vi "main(Test DQMH modules).vi"() -> ()   [LabVIEW 2018, in "Application.lvlib"] (continued)
        n3743 = Flush Queue(queue=w8192) -> (queue out=w8184:refnum<queue>)  [unwired: 1 in, 2 out]
        n3744 = Decrement(x=w8179) -> (x-1=w8183:i32)
        n3745 = Index Array(array=w8180, index=w8183) -> (element=w8181:refnum<vi>)
        n3746 = property class="ColBox"(reference=w8181, "Value"=u32 10000536 ("DRV 1")) -> ()  [unwired: 1 in, 2 out]
        n3747 = To Variant(anything=bool[] [FALSE, TRUE, FALSE, FALSE, FALSE, FALSE]) -> (Variant=w8209:variant)
        n3748 = To Variant(anything=T6."demux1_10_channel7" ("demux1_10(x6)_encode")) -> (Variant=w8213:variant)
        n3749 = To Variant(anything=T4."mux6_1_channel2_3" ("mux6_1(3wires)_encode")) -> (Variant=w8216:variant)
        n3750 = To Variant(anything=T5."mux10_1_channel7" ("mux10_1(x6)_encode")) -> (Variant=w8218:variant)
        n3751 = Bundle By Name(cluster=w8212, "command"="MEAS.mux10-1", "command data"=w8218) -> (w8207:T11)
        n3752 = Bundle By Name(cluster=w8212, "command"="MEAS.mux6_1", "command data"=w8216) -> (w8206:T11)
        n3753 = Bundle By Name(cluster=w8212, "command"="MEAS.demux1-10", "command data"=w8213) -> (w8205:T11)
        n3754 = Bundle By Name(cluster=w8212, "command"="MEAS.eMIC", "command data"=w8209) -> (w8204:T11)
        n3755 = Bundle By Name(cluster=w8212, "command"="MEAS.AllRelaysOFF") -> (w8208:T11)
        n3756 = Build Array(w8208, w8207, w8206, w8205, w8204) -> (w8199:T11[])
        n3757 = Bundle By Name(cluster=w8187, "command"="MEAS.requestAC", "command data"=w8179) -> (w8200:T11)
        n3758 = Bundle By Name(cluster=w8187, "command"="Apps.WaitForEvent", "command data"=w8179) -> (w8186:T11)
        n3759 = Bundle By Name(cluster=w8187, "command"="MEAS.DMM dual read") -> (w8201:T11)
        n3760 = Bundle By Name(cluster=w8187, "command"="Apps.UI Update 1") -> (w8188:T11)
        n3761 = Build Array(w8201, w8200, w8186, w8188) -> (w8198:T11[])
        n3762 = Build Array (concatenate)(w8199, w8198) -> (w8197:T11[])
        n3763 = for {
          tunnel: w8197 -> [w8234] mode=indexing
          tunnel: w8184 -> [w8235]
          tunnel: [w8231] -> w8195 mode=indexing
          n3764 = Unbundle By Name(w8234) -> ("command"=w8233:string, "command data"=w8232:variant)
          n3765 = call "App enquece.vi"("command data"=w8232, "command"=w8233, "queue in"=w8235) -> ("error out"=w8231:errorcluster)  [unwired: 7 in, 1 out]
        }
        n3766 = Merge Errors(w8196, w8195) -> (w8194:errorcluster)
      }
      frame "Test DRV 39A" {
        w8243 = T11 {"command"="", "command data"=variant} ("element")
        w8236 = 39 ("DUT index(0-59)")
        w8269 = T11 {"command"="", "command data"=variant} ("element")
        n3767 = disable-structure shown="LOGGING==TRUE" {
          disable-tunnel: w8247 -> [w8284 _]
          frame condition #0 (active) {
            n3768 = Empty String/Path?(string/path=w8284) -> (empty?=w8287:bool)
            n3769 = Select(t="Quece timeout", s=w8287, f=w8284) -> (s? t:f=w8283:string)
            n3770 = call "string log (SubVI).vi"("Enum"=enum16{"Init", "Log", "Read"}."Log", "state Name"=w8283) -> ()  [unwired: 8 in, 2 out]
          }
          frame condition #1 {
          }
        }
        n3771 = Flush Queue(queue=w8248) -> (queue out=w8249:refnum<queue>)  [unwired: 1 in, 2 out]
        n3772 = Decrement(x=w8236) -> (x-1=w8240:i32)
        n3773 = Index Array(array=w8237, index=w8240) -> (element=w8238:refnum<vi>)
        n3774 = property class="ColBox"(reference=w8238, "Value"=u32 10000536 ("DRV 1")) -> ()  [unwired: 1 in, 2 out]
        n3775 = To Variant(anything=bool[] [FALSE, FALSE, TRUE, FALSE, FALSE, FALSE]) -> (Variant=w8266:variant)
        n3776 = To Variant(anything=T6."demux1_10_channel7" ("demux1_10(x6)_encode")) -> (Variant=w8270:variant)
        n3777 = To Variant(anything=T4."mux6_1_channel3_3" ("mux6_1(3wires)_encode")) -> (Variant=w8273:variant)
        n3778 = To Variant(anything=T5."mux10_1_channel7" ("mux10_1(x6)_encode")) -> (Variant=w8275:variant)
        n3779 = Bundle By Name(cluster=w8269, "command"="MEAS.mux10-1", "command data"=w8275) -> (w8264:T11)
        n3780 = Bundle By Name(cluster=w8269, "command"="MEAS.mux6_1", "command data"=w8273) -> (w8263:T11)
        n3781 = Bundle By Name(cluster=w8269, "command"="MEAS.demux1-10", "command data"=w8270) -> (w8262:T11)
        n3782 = Bundle By Name(cluster=w8269, "command"="MEAS.eMIC", "command data"=w8266) -> (w8261:T11)
        n3783 = Bundle By Name(cluster=w8269, "command"="MEAS.AllRelaysOFF") -> (w8265:T11)
        n3784 = Build Array(w8265, w8264, w8263, w8262, w8261) -> (w8256:T11[])
        n3785 = Bundle By Name(cluster=w8243, "command"="MEAS.requestAC", "command data"=w8236) -> (w8257:T11)
        n3786 = Bundle By Name(cluster=w8243, "command"="Apps.WaitForEvent", "command data"=w8236) -> (w8242:T11)
        n3787 = Bundle By Name(cluster=w8243, "command"="MEAS.DMM dual read") -> (w8258:T11)
        n3788 = Bundle By Name(cluster=w8243, "command"="Apps.UI Update 1") -> (w8244:T11)
        n3789 = Build Array(w8258, w8257, w8242, w8244) -> (w8255:T11[])
        n3790 = Build Array (concatenate)(w8256, w8255) -> (w8254:T11[])
        n3791 = for {
          tunnel: w8254 -> [w8291] mode=indexing
          tunnel: w8249 -> [w8292]
          tunnel: [w8288] -> w8252 mode=indexing
          n3792 = Unbundle By Name(w8291) -> ("command"=w8290:string, "command data"=w8289:variant)
          n3793 = call "App enquece.vi"("command data"=w8289, "command"=w8290, "queue in"=w8292) -> ("error out"=w8288:errorcluster)  [unwired: 7 in, 1 out]
        }
        n3794 = Merge Errors(w8253, w8252) -> (w8251:errorcluster)
      }
      frame "Test DRV 40A" {
        w8300 = T11 {"command"="", "command data"=variant} ("element")
        w8293 = 40 ("DUT index(0-59)")
        w8326 = T11 {"command"="", "command data"=variant} ("element")
        n3795 = disable-structure shown="LOGGING==TRUE" {
          disable-tunnel: w8304 -> [w8341 _]
          frame condition #0 (active) {
            n3796 = Empty String/Path?(string/path=w8341) -> (empty?=w8344:bool)
            n3797 = Select(t="Quece timeout", s=w8344, f=w8341) -> (s? t:f=w8340:string)
            n3798 = call "string log (SubVI).vi"("Enum"=enum16{"Init", "Log", "Read"}."Log", "state Name"=w8340) -> ()  [unwired: 8 in, 2 out]
          }
          frame condition #1 {
          }
        }
        n3799 = Flush Queue(queue=w8305) -> (queue out=w8306:refnum<queue>)  [unwired: 1 in, 2 out]
        n3800 = Decrement(x=w8293) -> (x-1=w8297:i32)
        n3801 = Index Array(array=w8294, index=w8297) -> (element=w8295:refnum<vi>)
        n3802 = property class="ColBox"(reference=w8295, "Value"=u32 10000536 ("DRV 1")) -> ()  [unwired: 1 in, 2 out]
        n3803 = To Variant(anything=bool[] [FALSE, FALSE, FALSE, TRUE, FALSE, FALSE]) -> (Variant=w8323:variant)
        n3804 = To Variant(anything=T6."demux1_10_channel7" ("demux1_10(x6)_encode")) -> (Variant=w8327:variant)
        n3805 = To Variant(anything=T4."mux6_1_channel4_3" ("mux6_1(3wires)_encode")) -> (Variant=w8330:variant)
        n3806 = To Variant(anything=T5."mux10_1_channel7" ("mux10_1(x6)_encode")) -> (Variant=w8332:variant)
        n3807 = Bundle By Name(cluster=w8326, "command"="MEAS.mux10-1", "command data"=w8332) -> (w8321:T11)
        n3808 = Bundle By Name(cluster=w8326, "command"="MEAS.mux6_1", "command data"=w8330) -> (w8320:T11)
        n3809 = Bundle By Name(cluster=w8326, "command"="MEAS.demux1-10", "command data"=w8327) -> (w8319:T11)
        n3810 = Bundle By Name(cluster=w8326, "command"="MEAS.eMIC", "command data"=w8323) -> (w8318:T11)
        n3811 = Bundle By Name(cluster=w8326, "command"="MEAS.AllRelaysOFF") -> (w8322:T11)
        n3812 = Build Array(w8322, w8321, w8320, w8319, w8318) -> (w8313:T11[])
        n3813 = Bundle By Name(cluster=w8300, "command"="MEAS.requestAC", "command data"=w8293) -> (w8314:T11)
        n3814 = Bundle By Name(cluster=w8300, "command"="Apps.WaitForEvent", "command data"=w8293) -> (w8299:T11)
        n3815 = Bundle By Name(cluster=w8300, "command"="MEAS.DMM dual read") -> (w8315:T11)
        n3816 = Bundle By Name(cluster=w8300, "command"="Apps.UI Update 1") -> (w8301:T11)
        n3817 = Build Array(w8315, w8314, w8299, w8301) -> (w8312:T11[])
        n3818 = Build Array (concatenate)(w8313, w8312) -> (w8311:T11[])
        n3819 = for {
          tunnel: w8311 -> [w8348] mode=indexing
          tunnel: w8306 -> [w8349]
          tunnel: [w8345] -> w8309 mode=indexing
          n3820 = Unbundle By Name(w8348) -> ("command"=w8347:string, "command data"=w8346:variant)
          n3821 = call "App enquece.vi"("command data"=w8346, "command"=w8347, "queue in"=w8349) -> ("error out"=w8345:errorcluster)  [unwired: 7 in, 1 out]
        }
        n3822 = Merge Errors(w8310, w8309) -> (w8308:errorcluster)
      }
      frame "Test DRV 41A" {
        w8357 = T11 {"command"="", "command data"=variant} ("element")
        w8350 = 41 ("DUT index(0-59)")
        w8383 = T11 {"command"="", "command data"=variant} ("element")
        n3823 = disable-structure shown="LOGGING==TRUE" {
          disable-tunnel: w8361 -> [w8398 _]
          frame condition #0 (active) {
            n3824 = Empty String/Path?(string/path=w8398) -> (empty?=w8401:bool)
            n3825 = Select(t="Quece timeout", s=w8401, f=w8398) -> (s? t:f=w8397:string)
            n3826 = call "string log (SubVI).vi"("Enum"=enum16{"Init", "Log", "Read"}."Log", "state Name"=w8397) -> ()  [unwired: 8 in, 2 out]
          }
          frame condition #1 {
          }
        }
        n3827 = Flush Queue(queue=w8362) -> (queue out=w8363:refnum<queue>)  [unwired: 1 in, 2 out]
        n3828 = Decrement(x=w8350) -> (x-1=w8354:i32)
        n3829 = Index Array(array=w8351, index=w8354) -> (element=w8352:refnum<vi>)
        n3830 = property class="ColBox"(reference=w8352, "Value"=u32 10000536 ("DRV 1")) -> ()  [unwired: 1 in, 2 out]
        n3831 = To Variant(anything=bool[] [FALSE, FALSE, FALSE, FALSE, TRUE, FALSE]) -> (Variant=w8380:variant)
        n3832 = To Variant(anything=T6."demux1_10_channel7" ("demux1_10(x6)_encode")) -> (Variant=w8384:variant)
        n3833 = To Variant(anything=T4."mux6_1_channel5_3" ("mux6_1(3wires)_encode")) -> (Variant=w8387:variant)
        n3834 = To Variant(anything=T5."mux10_1_channel7" ("mux10_1(x6)_encode")) -> (Variant=w8389:variant)
        n3835 = Bundle By Name(cluster=w8383, "command"="MEAS.mux10-1", "command data"=w8389) -> (w8378:T11)
        n3836 = Bundle By Name(cluster=w8383, "command"="MEAS.mux6_1", "command data"=w8387) -> (w8377:T11)
        n3837 = Bundle By Name(cluster=w8383, "command"="MEAS.demux1-10", "command data"=w8384) -> (w8376:T11)
        n3838 = Bundle By Name(cluster=w8383, "command"="MEAS.eMIC", "command data"=w8380) -> (w8375:T11)
        n3839 = Bundle By Name(cluster=w8383, "command"="MEAS.AllRelaysOFF") -> (w8379:T11)
        n3840 = Build Array(w8379, w8378, w8377, w8376, w8375) -> (w8370:T11[])
        n3841 = Bundle By Name(cluster=w8357, "command"="MEAS.requestAC", "command data"=w8350) -> (w8371:T11)
        n3842 = Bundle By Name(cluster=w8357, "command"="Apps.WaitForEvent", "command data"=w8350) -> (w8356:T11)
        n3843 = Bundle By Name(cluster=w8357, "command"="MEAS.DMM dual read") -> (w8372:T11)
        n3844 = Bundle By Name(cluster=w8357, "command"="Apps.UI Update 1") -> (w8358:T11)
        n3845 = Build Array(w8372, w8371, w8356, w8358) -> (w8369:T11[])
        n3846 = Build Array (concatenate)(w8370, w8369) -> (w8368:T11[])
        n3847 = for {
          tunnel: w8368 -> [w8405] mode=indexing
          tunnel: w8363 -> [w8406]
          tunnel: [w8402] -> w8366 mode=indexing
          n3848 = Unbundle By Name(w8405) -> ("command"=w8404:string, "command data"=w8403:variant)
          n3849 = call "App enquece.vi"("command data"=w8403, "command"=w8404, "queue in"=w8406) -> ("error out"=w8402:errorcluster)  [unwired: 7 in, 1 out]
        }
        n3850 = Merge Errors(w8367, w8366) -> (w8365:errorcluster)
      }
      frame "Test DRV 42A" {
        w8414 = T11 {"command"="", "command data"=variant} ("element")
        w8407 = 42 ("DUT index(0-59)")
        w8440 = T11 {"command"="", "command data"=variant} ("element")
        n3851 = disable-structure shown="LOGGING==TRUE" {
          disable-tunnel: w8418 -> [w8455 _]
          frame condition #0 (active) {
            n3852 = Empty String/Path?(string/path=w8455) -> (empty?=w8458:bool)
            n3853 = Select(t="Quece timeout", s=w8458, f=w8455) -> (s? t:f=w8454:string)
            n3854 = call "string log (SubVI).vi"("Enum"=enum16{"Init", "Log", "Read"}."Log", "state Name"=w8454) -> ()  [unwired: 8 in, 2 out]
          }
          frame condition #1 {
          }
        }
        n3855 = Flush Queue(queue=w8419) -> (queue out=w8420:refnum<queue>)  [unwired: 1 in, 2 out]
        n3856 = Decrement(x=w8407) -> (x-1=w8411:i32)
        n3857 = Index Array(array=w8408, index=w8411) -> (element=w8409:refnum<vi>)
        n3858 = property class="ColBox"(reference=w8409, "Value"=u32 10000536 ("DRV 1")) -> ()  [unwired: 1 in, 2 out]
        n3859 = To Variant(anything=bool[] [FALSE, FALSE, FALSE, FALSE, FALSE, TRUE]) -> (Variant=w8437:variant)
        n3860 = To Variant(anything=T6."demux1_10_channel7" ("demux1_10(x6)_encode")) -> (Variant=w8441:variant)
        n3861 = To Variant(anything=T4."mux6_1_channel6_3" ("mux6_1(3wires)_encode")) -> (Variant=w8444:variant)
        n3862 = To Variant(anything=T5."mux10_1_channel7" ("mux10_1(x6)_encode")) -> (Variant=w8446:variant)
        n3863 = Bundle By Name(cluster=w8440, "command"="MEAS.mux10-1", "command data"=w8446) -> (w8435:T11)
        n3864 = Bundle By Name(cluster=w8440, "command"="MEAS.mux6_1", "command data"=w8444) -> (w8434:T11)
        n3865 = Bundle By Name(cluster=w8440, "command"="MEAS.demux1-10", "command data"=w8441) -> (w8433:T11)
        n3866 = Bundle By Name(cluster=w8440, "command"="MEAS.eMIC", "command data"=w8437) -> (w8432:T11)
        n3867 = Bundle By Name(cluster=w8440, "command"="MEAS.AllRelaysOFF") -> (w8436:T11)
        n3868 = Build Array(w8436, w8435, w8434, w8433, w8432) -> (w8427:T11[])
        n3869 = Bundle By Name(cluster=w8414, "command"="MEAS.requestAC", "command data"=w8407) -> (w8428:T11)
        n3870 = Bundle By Name(cluster=w8414, "command"="Apps.WaitForEvent", "command data"=w8407) -> (w8413:T11)
        n3871 = Bundle By Name(cluster=w8414, "command"="MEAS.DMM dual read") -> (w8429:T11)
        n3872 = Bundle By Name(cluster=w8414, "command"="Apps.UI Update 1") -> (w8415:T11)
        n3873 = Build Array(w8429, w8428, w8413, w8415) -> (w8426:T11[])
        n3874 = Build Array (concatenate)(w8427, w8426) -> (w8425:T11[])
        n3875 = for {
          tunnel: w8425 -> [w8462] mode=indexing
          tunnel: w8420 -> [w8463]
          tunnel: [w8459] -> w8423 mode=indexing
          n3876 = Unbundle By Name(w8462) -> ("command"=w8461:string, "command data"=w8460:variant)
          n3877 = call "App enquece.vi"("command data"=w8460, "command"=w8461, "queue in"=w8463) -> ("error out"=w8459:errorcluster)  [unwired: 7 in, 1 out]
        }
        n3878 = Merge Errors(w8424, w8423) -> (w8422:errorcluster)
      }
      frame "Test DRV 43A" {
        w8471 = T11 {"command"="", "command data"=variant} ("element")
        w8464 = 43 ("DUT index(0-59)")
        w8497 = T11 {"command"="", "command data"=variant} ("element")
        n3879 = disable-structure shown="LOGGING==TRUE" {
          disable-tunnel: w8475 -> [w8512 _]
          frame condition #0 (active) {
            n3880 = Empty String/Path?(string/path=w8512) -> (empty?=w8515:bool)
            n3881 = Select(t="Quece timeout", s=w8515, f=w8512) -> (s? t:f=w8511:string)
            n3882 = call "string log (SubVI).vi"("Enum"=enum16{"Init", "Log", "Read"}."Log", "state Name"=w8511) -> ()  [unwired: 8 in, 2 out]
          }
          frame condition #1 {
          }
        }
        n3883 = Flush Queue(queue=w8476) -> (queue out=w8477:refnum<queue>)  [unwired: 1 in, 2 out]
        n3884 = Decrement(x=w8464) -> (x-1=w8468:i32)
        n3885 = Index Array(array=w8465, index=w8468) -> (element=w8466:refnum<vi>)
        n3886 = property class="ColBox"(reference=w8466, "Value"=u32 10000536 ("DRV 1")) -> ()  [unwired: 1 in, 2 out]
        n3887 = To Variant(anything=bool[] [TRUE, FALSE, FALSE, FALSE, FALSE, FALSE]) -> (Variant=w8494:variant)
        n3888 = To Variant(anything=T6."demux1_10_channel8" ("demux1_10(x6)_encode")) -> (Variant=w8498:variant)
        n3889 = To Variant(anything=T4."mux6_1_channel1_3" ("mux6_1(3wires)_encode")) -> (Variant=w8501:variant)
        n3890 = To Variant(anything=T5."mux10_1_channel8" ("mux10_1(x6)_encode")) -> (Variant=w8503:variant)
        n3891 = Bundle By Name(cluster=w8497, "command"="MEAS.mux10-1", "command data"=w8503) -> (w8492:T11)
        n3892 = Bundle By Name(cluster=w8497, "command"="MEAS.mux6_1", "command data"=w8501) -> (w8491:T11)
        n3893 = Bundle By Name(cluster=w8497, "command"="MEAS.demux1-10", "command data"=w8498) -> (w8490:T11)
        n3894 = Bundle By Name(cluster=w8497, "command"="MEAS.eMIC", "command data"=w8494) -> (w8489:T11)
        n3895 = Bundle By Name(cluster=w8497, "command"="MEAS.AllRelaysOFF") -> (w8493:T11)
        n3896 = Build Array(w8493, w8492, w8491, w8490, w8489) -> (w8484:T11[])
        n3897 = Bundle By Name(cluster=w8471, "command"="MEAS.requestAC", "command data"=w8464) -> (w8485:T11)
        n3898 = Bundle By Name(cluster=w8471, "command"="Apps.WaitForEvent", "command data"=w8464) -> (w8470:T11)
        n3899 = Bundle By Name(cluster=w8471, "command"="MEAS.DMM dual read") -> (w8486:T11)
        n3900 = Bundle By Name(cluster=w8471, "command"="Apps.UI Update 1") -> (w8472:T11)
        n3901 = Build Array(w8486, w8485, w8470, w8472) -> (w8483:T11[])
        n3902 = Build Array (concatenate)(w8484, w8483) -> (w8482:T11[])
        n3903 = for {
          tunnel: w8482 -> [w8519] mode=indexing
          tunnel: w8477 -> [w8520]
          tunnel: [w8516] -> w8480 mode=indexing
          n3904 = Unbundle By Name(w8519) -> ("command"=w8518:string, "command data"=w8517:variant)
          n3905 = call "App enquece.vi"("command data"=w8517, "command"=w8518, "queue in"=w8520) -> ("error out"=w8516:errorcluster)  [unwired: 7 in, 1 out]
        }
        n3906 = Merge Errors(w8481, w8480) -> (w8479:errorcluster)
      }
      frame "Test DRV 44A" {
        w8528 = T11 {"command"="", "command data"=variant} ("element")
        w8524 = 44 ("DUT index(0-59)")
        w8554 = T11 {"command"="", "command data"=variant} ("element")
        n3907 = disable-structure shown="LOGGING==TRUE" {
          disable-tunnel: w8532 -> [w8569 _]
          frame condition #0 (active) {
            n3908 = Empty String/Path?(string/path=w8569) -> (empty?=w8572:bool)
            n3909 = Select(t="Quece timeout", s=w8572, f=w8569) -> (s? t:f=w8568:string)
            n3910 = call "string log (SubVI).vi"("Enum"=enum16{"Init", "Log", "Read"}."Log", "state Name"=w8568) -> ()  [unwired: 8 in, 2 out]
          }
          frame condition #1 {
          }
        }
        n3911 = Flush Queue(queue=w8533) -> (queue out=w8534:refnum<queue>)  [unwired: 1 in, 2 out]
        n3912 = Decrement(x=w8524) -> (x-1=w8525:i32)
        n3913 = Index Array(array=w8523, index=w8525) -> (element=w8521:refnum<vi>)
        n3914 = property class="ColBox"(reference=w8521, "Value"=u32 10000536 ("DRV 1")) -> ()  [unwired: 1 in, 2 out]
        n3915 = To Variant(anything=bool[] [FALSE, TRUE, FALSE, FALSE, FALSE, FALSE]) -> (Variant=w8551:variant)
        n3916 = To Variant(anything=T6."demux1_10_channel8" ("demux1_10(x6)_encode")) -> (Variant=w8555:variant)
        n3917 = To Variant(anything=T4."mux6_1_channel2_3" ("mux6_1(3wires)_encode")) -> (Variant=w8558:variant)
        n3918 = To Variant(anything=T5."mux10_1_channel8" ("mux10_1(x6)_encode")) -> (Variant=w8560:variant)
        n3919 = Bundle By Name(cluster=w8554, "command"="MEAS.mux10-1", "command data"=w8560) -> (w8549:T11)
        n3920 = Bundle By Name(cluster=w8554, "command"="MEAS.mux6_1", "command data"=w8558) -> (w8548:T11)
        n3921 = Bundle By Name(cluster=w8554, "command"="MEAS.demux1-10", "command data"=w8555) -> (w8547:T11)
        n3922 = Bundle By Name(cluster=w8554, "command"="MEAS.eMIC", "command data"=w8551) -> (w8546:T11)
        n3923 = Bundle By Name(cluster=w8554, "command"="MEAS.AllRelaysOFF") -> (w8550:T11)
        n3924 = Build Array(w8550, w8549, w8548, w8547, w8546) -> (w8541:T11[])
        n3925 = Bundle By Name(cluster=w8528, "command"="MEAS.requestAC", "command data"=w8524) -> (w8542:T11)
        n3926 = Bundle By Name(cluster=w8528, "command"="Apps.WaitForEvent", "command data"=w8524) -> (w8527:T11)
        n3927 = Bundle By Name(cluster=w8528, "command"="MEAS.DMM dual read") -> (w8543:T11)
        n3928 = Bundle By Name(cluster=w8528, "command"="Apps.UI Update 1") -> (w8529:T11)
        n3929 = Build Array(w8543, w8542, w8527, w8529) -> (w8540:T11[])
        n3930 = Build Array (concatenate)(w8541, w8540) -> (w8539:T11[])
        n3931 = for {
          tunnel: w8539 -> [w8576] mode=indexing
          tunnel: w8534 -> [w8577]
          tunnel: [w8573] -> w8537 mode=indexing
          n3932 = Unbundle By Name(w8576) -> ("command"=w8575:string, "command data"=w8574:variant)
          n3933 = call "App enquece.vi"("command data"=w8574, "command"=w8575, "queue in"=w8577) -> ("error out"=w8573:errorcluster)  [unwired: 7 in, 1 out]
        }
        n3934 = Merge Errors(w8538, w8537) -> (w8536:errorcluster)
      }
      frame "Test DRV 45A" {
        w8585 = T11 {"command"="", "command data"=variant} ("element")
        w8578 = 45 ("DUT index(0-59)")
        w8611 = T11 {"command"="", "command data"=variant} ("element")
        n3935 = disable-structure shown="LOGGING==TRUE" {
          disable-tunnel: w8589 -> [w8626 _]
          frame condition #0 (active) {
            n3936 = Empty String/Path?(string/path=w8626) -> (empty?=w8629:bool)
            n3937 = Select(t="Quece timeout", s=w8629, f=w8626) -> (s? t:f=w8625:string)
            n3938 = call "string log (SubVI).vi"("Enum"=enum16{"Init", "Log", "Read"}."Log", "state Name"=w8625) -> ()  [unwired: 8 in, 2 out]
          }
          frame condition #1 {
          }
        }
        n3939 = Flush Queue(queue=w8590) -> (queue out=w8591:refnum<queue>)  [unwired: 1 in, 2 out]
        n3940 = Decrement(x=w8578) -> (x-1=w8582:i32)
        n3941 = Index Array(array=w8579, index=w8582) -> (element=w8580:refnum<vi>)
        n3942 = property class="ColBox"(reference=w8580, "Value"=u32 10000536 ("DRV 1")) -> ()  [unwired: 1 in, 2 out]
        n3943 = To Variant(anything=bool[] [FALSE, FALSE, TRUE, FALSE, FALSE, FALSE]) -> (Variant=w8608:variant)
        n3944 = To Variant(anything=T6."demux1_10_channel8" ("demux1_10(x6)_encode")) -> (Variant=w8612:variant)
        n3945 = To Variant(anything=T4."mux6_1_channel3_3" ("mux6_1(3wires)_encode")) -> (Variant=w8615:variant)
        n3946 = To Variant(anything=T5."mux10_1_channel8" ("mux10_1(x6)_encode")) -> (Variant=w8617:variant)
        n3947 = Bundle By Name(cluster=w8611, "command"="MEAS.mux10-1", "command data"=w8617) -> (w8606:T11)
        n3948 = Bundle By Name(cluster=w8611, "command"="MEAS.mux6_1", "command data"=w8615) -> (w8605:T11)
        n3949 = Bundle By Name(cluster=w8611, "command"="MEAS.demux1-10", "command data"=w8612) -> (w8604:T11)
        n3950 = Bundle By Name(cluster=w8611, "command"="MEAS.eMIC", "command data"=w8608) -> (w8603:T11)
        n3951 = Bundle By Name(cluster=w8611, "command"="MEAS.AllRelaysOFF") -> (w8607:T11)
        n3952 = Build Array(w8607, w8606, w8605, w8604, w8603) -> (w8598:T11[])
        n3953 = Bundle By Name(cluster=w8585, "command"="MEAS.requestAC", "command data"=w8578) -> (w8599:T11)
        n3954 = Bundle By Name(cluster=w8585, "command"="Apps.WaitForEvent", "command data"=w8578) -> (w8584:T11)
        n3955 = Bundle By Name(cluster=w8585, "command"="MEAS.DMM dual read") -> (w8600:T11)
        n3956 = Bundle By Name(cluster=w8585, "command"="Apps.UI Update 1") -> (w8586:T11)
        n3957 = Build Array(w8600, w8599, w8584, w8586) -> (w8597:T11[])
        n3958 = Build Array (concatenate)(w8598, w8597) -> (w8596:T11[])
        n3959 = for {
          tunnel: w8596 -> [w8633] mode=indexing
          tunnel: w8591 -> [w8634]
          tunnel: [w8630] -> w8594 mode=indexing
          n3960 = Unbundle By Name(w8633) -> ("command"=w8632:string, "command data"=w8631:variant)
          n3961 = call "App enquece.vi"("command data"=w8631, "command"=w8632, "queue in"=w8634) -> ("error out"=w8630:errorcluster)  [unwired: 7 in, 1 out]
        }
        n3962 = Merge Errors(w8595, w8594) -> (w8593:errorcluster)
      }
      frame "Test DRV 46A" {
        w8642 = T11 {"command"="", "command data"=variant} ("element")
        w8636 = 46 ("DUT index(0-59)")
        w8668 = T11 {"command"="", "command data"=variant} ("element")
        n3963 = disable-structure shown="LOGGING==TRUE" {
          disable-tunnel: w8646 -> [w8683 _]
          frame condition #0 (active) {
            n3964 = Empty String/Path?(string/path=w8683) -> (empty?=w8686:bool)
            n3965 = Select(t="Quece timeout", s=w8686, f=w8683) -> (s? t:f=w8682:string)
            n3966 = call "string log (SubVI).vi"("Enum"=enum16{"Init", "Log", "Read"}."Log", "state Name"=w8682) -> ()  [unwired: 8 in, 2 out]
          }
          frame condition #1 {
          }
        }
        n3967 = Decrement(x=w8636) -> (x-1=w8639:i32)
        n3968 = Flush Queue(queue=w8647) -> (queue out=w8648:refnum<queue>)  [unwired: 1 in, 2 out]
        n3969 = Index Array(array=w8635, index=w8639) -> (element=w8637:refnum<vi>)
        n3970 = property class="ColBox"(reference=w8637, "Value"=u32 10000536 ("DRV 1")) -> ()  [unwired: 1 in, 2 out]
        n3971 = To Variant(anything=bool[] [FALSE, FALSE, TRUE, FALSE, FALSE, FALSE]) -> (Variant=w8665:variant)
        n3972 = To Variant(anything=T6."demux1_10_channel8" ("demux1_10(x6)_encode")) -> (Variant=w8669:variant)
        n3973 = To Variant(anything=T4."mux6_1_channel3_3" ("mux6_1(3wires)_encode")) -> (Variant=w8672:variant)
        n3974 = To Variant(anything=T5."mux10_1_channel8" ("mux10_1(x6)_encode")) -> (Variant=w8674:variant)
        n3975 = Bundle By Name(cluster=w8668, "command"="MEAS.mux10-1", "command data"=w8674) -> (w8663:T11)
        n3976 = Bundle By Name(cluster=w8668, "command"="MEAS.mux6_1", "command data"=w8672) -> (w8662:T11)
        n3977 = Bundle By Name(cluster=w8668, "command"="MEAS.demux1-10", "command data"=w8669) -> (w8661:T11)
        n3978 = Bundle By Name(cluster=w8668, "command"="MEAS.eMIC", "command data"=w8665) -> (w8660:T11)
        n3979 = Bundle By Name(cluster=w8668, "command"="MEAS.AllRelaysOFF") -> (w8664:T11)
        n3980 = Build Array(w8664, w8663, w8662, w8661, w8660) -> (w8655:T11[])
        n3981 = Bundle By Name(cluster=w8642, "command"="MEAS.requestAC", "command data"=w8636) -> (w8656:T11)
        n3982 = Bundle By Name(cluster=w8642, "command"="Apps.WaitForEvent", "command data"=w8636) -> (w8641:T11)
        n3983 = Bundle By Name(cluster=w8642, "command"="MEAS.DMM dual read") -> (w8657:T11)
        n3984 = Bundle By Name(cluster=w8642, "command"="Apps.UI Update 1") -> (w8643:T11)
        n3985 = Build Array(w8657, w8656, w8641, w8643) -> (w8654:T11[])
        n3986 = Build Array (concatenate)(w8655, w8654) -> (w8653:T11[])
        n3987 = for {
          tunnel: w8653 -> [w8690] mode=indexing
          tunnel: w8648 -> [w8691]
          tunnel: [w8687] -> w8651 mode=indexing
          n3988 = Unbundle By Name(w8690) -> ("command"=w8689:string, "command data"=w8688:variant)
          n3989 = call "App enquece.vi"("command data"=w8688, "command"=w8689, "queue in"=w8691) -> ("error out"=w8687:errorcluster)  [unwired: 7 in, 1 out]
        }
        n3990 = Merge Errors(w8652, w8651) -> (w8650:errorcluster)
      }
      frame "Test DRV 47A" {
        w8701 = T11 {"command"="", "command data"=variant} ("element")
        w8692 = 47 ("DUT index(0-59)")
        w8725 = T11 {"command"="", "command data"=variant} ("element")
        n3991 = disable-structure shown="LOGGING==TRUE" {
          disable-tunnel: w8705 -> [w8740 _]
          frame condition #0 (active) {
            n3992 = Empty String/Path?(string/path=w8740) -> (empty?=w8743:bool)
            n3993 = Select(t="Quece timeout", s=w8743, f=w8740) -> (s? t:f=w8739:string)
            n3994 = call "string log (SubVI).vi"("Enum"=enum16{"Init", "Log", "Read"}."Log", "state Name"=w8739) -> ()  [unwired: 8 in, 2 out]
          }
          frame condition #1 {
          }
        }
        n3995 = Decrement(x=w8692) -> (x-1=w8696:i32)
        n3996 = Flush Queue(queue=w8706) -> (queue out=w8707:refnum<queue>)  [unwired: 1 in, 2 out]
        n3997 = Index Array(array=w8693, index=w8696) -> (element=w8694:refnum<vi>)
        n3998 = property class="ColBox"(reference=w8694, "Value"=u32 10000536 ("DRV 1")) -> ()  [unwired: 1 in, 2 out]
        n3999 = To Variant(anything=bool[] [FALSE, FALSE, FALSE, FALSE, TRUE, FALSE]) -> (Variant=w8722:variant)
        n4000 = To Variant(anything=T6."demux1_10_channel8" ("demux1_10(x6)_encode")) -> (Variant=w8726:variant)
        n4001 = To Variant(anything=T4."mux6_1_channel5_3" ("mux6_1(3wires)_encode")) -> (Variant=w8729:variant)
        n4002 = To Variant(anything=T5."mux10_1_channel8" ("mux10_1(x6)_encode")) -> (Variant=w8731:variant)
        n4003 = Bundle By Name(cluster=w8725, "command"="MEAS.mux10-1", "command data"=w8731) -> (w8720:T11)
        n4004 = Bundle By Name(cluster=w8725, "command"="MEAS.mux6_1", "command data"=w8729) -> (w8719:T11)
        n4005 = Bundle By Name(cluster=w8725, "command"="MEAS.demux1-10", "command data"=w8726) -> (w8718:T11)
        n4006 = Bundle By Name(cluster=w8725, "command"="MEAS.eMIC", "command data"=w8722) -> (w8717:T11)
        n4007 = Bundle By Name(cluster=w8725, "command"="MEAS.AllRelaysOFF") -> (w8721:T11)
        n4008 = Build Array(w8721, w8720, w8719, w8718, w8717) -> (w8712:T11[])
        n4009 = Bundle By Name(cluster=w8701, "command"="MEAS.requestAC", "command data"=w8692) -> (w8713:T11)
        n4010 = Bundle By Name(cluster=w8701, "command"="Apps.WaitForEvent", "command data"=w8692) -> (w8700:T11)
        n4011 = Bundle By Name(cluster=w8701, "command"="Apps.UI Update 1") -> (w8702:T11)
        n4012 = Bundle By Name(cluster=w8701, "command"="MEAS.DMM dual read") -> (w8714:T11)
        n4013 = Build Array(w8714, w8713, w8700, w8702) -> (w8711:T11[])
        n4014 = Build Array (concatenate)(w8712, w8711) -> (w8710:T11[])
        n4015 = for {
          tunnel: w8710 -> [w8747] mode=indexing
          tunnel: w8707 -> [w8748]
          tunnel: [w8744] -> w8709 mode=indexing
          n4016 = Unbundle By Name(w8747) -> ("command"=w8746:string, "command data"=w8745:variant)
          n4017 = call "App enquece.vi"("command data"=w8745, "command"=w8746, "queue in"=w8748) -> ("error out"=w8744:errorcluster)  [unwired: 7 in, 1 out]
        }
        n4018 = Merge Errors(w8697, w8709) -> (w8708:errorcluster)
      }
      frame "Test DRV 48A" {
        w8756 = T11 {"command"="", "command data"=variant} ("element")
        w8750 = 48 ("DUT index(0-59)")
        w8782 = T11 {"command"="", "command data"=variant} ("element")
        n4019 = disable-structure shown="LOGGING==TRUE" {
          disable-tunnel: w8760 -> [w8797 _]
          frame condition #0 (active) {
            n4020 = Empty String/Path?(string/path=w8797) -> (empty?=w8800:bool)
            n4021 = Select(t="Quece timeout", s=w8800, f=w8797) -> (s? t:f=w8796:string)
            n4022 = call "string log (SubVI).vi"("Enum"=enum16{"Init", "Log", "Read"}."Log", "state Name"=w8796) -> ()  [unwired: 8 in, 2 out]
          }
          frame condition #1 {
          }
        }
        n4023 = Decrement(x=w8750) -> (x-1=w8753:i32)
        n4024 = Flush Queue(queue=w8761) -> (queue out=w8762:refnum<queue>)  [unwired: 1 in, 2 out]
        n4025 = Index Array(array=w8751, index=w8753) -> (element=w8749:refnum<vi>)
        n4026 = property class="ColBox"(reference=w8749, "Value"=u32 10000536 ("DRV 1")) -> ()  [unwired: 1 in, 2 out]
        n4027 = To Variant(anything=bool[] [FALSE, FALSE, FALSE, FALSE, FALSE, TRUE]) -> (Variant=w8779:variant)
        n4028 = To Variant(anything=T6."demux1_10_channel8" ("demux1_10(x6)_encode")) -> (Variant=w8783:variant)
        n4029 = To Variant(anything=T4."mux6_1_channel6_3" ("mux6_1(3wires)_encode")) -> (Variant=w8786:variant)
        n4030 = To Variant(anything=T5."mux10_1_channel8" ("mux10_1(x6)_encode")) -> (Variant=w8788:variant)
        n4031 = Bundle By Name(cluster=w8782, "command"="MEAS.mux10-1", "command data"=w8788) -> (w8777:T11)
        n4032 = Bundle By Name(cluster=w8782, "command"="MEAS.mux6_1", "command data"=w8786) -> (w8776:T11)
        n4033 = Bundle By Name(cluster=w8782, "command"="MEAS.demux1-10", "command data"=w8783) -> (w8775:T11)
        n4034 = Bundle By Name(cluster=w8782, "command"="MEAS.eMIC", "command data"=w8779) -> (w8774:T11)
        n4035 = Bundle By Name(cluster=w8782, "command"="MEAS.AllRelaysOFF") -> (w8778:T11)
        n4036 = Build Array(w8778, w8777, w8776, w8775, w8774) -> (w8769:T11[])
        n4037 = Bundle By Name(cluster=w8756, "command"="MEAS.requestAC", "command data"=w8750) -> (w8770:T11)
        n4038 = Bundle By Name(cluster=w8756, "command"="Apps.WaitForEvent", "command data"=w8750) -> (w8755:T11)
        n4039 = Bundle By Name(cluster=w8756, "command"="MEAS.DMM dual read") -> (w8771:T11)
        n4040 = Bundle By Name(cluster=w8756, "command"="Apps.UI Update 1") -> (w8757:T11)
        n4041 = Build Array(w8771, w8770, w8755, w8757) -> (w8768:T11[])
        n4042 = Build Array (concatenate)(w8769, w8768) -> (w8767:T11[])
        n4043 = for {
          tunnel: w8767 -> [w8804] mode=indexing
          tunnel: w8762 -> [w8805]
          tunnel: [w8801] -> w8765 mode=indexing
          n4044 = Unbundle By Name(w8804) -> ("command"=w8803:string, "command data"=w8802:variant)
          n4045 = call "App enquece.vi"("command data"=w8802, "command"=w8803, "queue in"=w8805) -> ("error out"=w8801:errorcluster)  [unwired: 7 in, 1 out]
        }
        n4046 = Merge Errors(w8766, w8765) -> (w8764:errorcluster)
      }
      frame "Test DRV 49A" {
        w8813 = T11 {"command"="", "command data"=variant} ("element")
        w8807 = 49 ("DUT index(0-59)")
        w8839 = T11 {"command"="", "command data"=variant} ("element")
        n4047 = disable-structure shown="LOGGING==TRUE" {
          disable-tunnel: w8817 -> [w8854 _]
          frame condition #0 (active) {
            n4048 = Empty String/Path?(string/path=w8854) -> (empty?=w8857:bool)
            n4049 = Select(t="Quece timeout", s=w8857, f=w8854) -> (s? t:f=w8853:string)
            n4050 = call "string log (SubVI).vi"("Enum"=enum16{"Init", "Log", "Read"}."Log", "state Name"=w8853) -> ()  [unwired: 8 in, 2 out]
          }
          frame condition #1 {
          }
        }
        n4051 = Flush Queue(queue=w8818) -> (queue out=w8819:refnum<queue>)  [unwired: 1 in, 2 out]
        n4052 = Decrement(x=w8807) -> (x-1=w8810:i32)
        n4053 = Index Array(array=w8808, index=w8810) -> (element=w8806:refnum<vi>)
        n4054 = property class="ColBox"(reference=w8806, "Value"=u32 10000536 ("DRV 1")) -> ()  [unwired: 1 in, 2 out]
        n4055 = To Variant(anything=bool[] [TRUE, FALSE, FALSE, FALSE, FALSE, FALSE]) -> (Variant=w8836:variant)
        n4056 = To Variant(anything=T6."demux1_10_channel9" ("demux1_10(x6)_encode")) -> (Variant=w8840:variant)
        n4057 = To Variant(anything=T4."mux6_1_channel1_3" ("mux6_1(3wires)_encode")) -> (Variant=w8843:variant)
        n4058 = To Variant(anything=T5."mux10_1_channel9" ("mux10_1(x6)_encode")) -> (Variant=w8845:variant)
        n4059 = Bundle By Name(cluster=w8839, "command"="MEAS.mux10-1", "command data"=w8845) -> (w8834:T11)
        n4060 = Bundle By Name(cluster=w8839, "command"="MEAS.mux6_1", "command data"=w8843) -> (w8833:T11)
        n4061 = Bundle By Name(cluster=w8839, "command"="MEAS.demux1-10", "command data"=w8840) -> (w8832:T11)
        n4062 = Bundle By Name(cluster=w8839, "command"="MEAS.eMIC", "command data"=w8836) -> (w8831:T11)
        n4063 = Bundle By Name(cluster=w8839, "command"="MEAS.AllRelaysOFF") -> (w8835:T11)
        n4064 = Build Array(w8835, w8834, w8833, w8832, w8831) -> (w8826:T11[])
        n4065 = Bundle By Name(cluster=w8813, "command"="MEAS.requestAC", "command data"=w8807) -> (w8827:T11)
        n4066 = Bundle By Name(cluster=w8813, "command"="Apps.WaitForEvent", "command data"=w8807) -> (w8812:T11)
        n4067 = Bundle By Name(cluster=w8813, "command"="MEAS.DMM dual read") -> (w8828:T11)
        n4068 = Bundle By Name(cluster=w8813, "command"="Apps.UI Update 1") -> (w8814:T11)
        n4069 = Build Array(w8828, w8827, w8812, w8814) -> (w8825:T11[])
        n4070 = Build Array (concatenate)(w8826, w8825) -> (w8824:T11[])
        n4071 = for {
          tunnel: w8824 -> [w8861] mode=indexing
          tunnel: w8819 -> [w8862]
          tunnel: [w8858] -> w8822 mode=indexing
          n4072 = Unbundle By Name(w8861) -> ("command"=w8860:string, "command data"=w8859:variant)
          n4073 = call "App enquece.vi"("command data"=w8859, "command"=w8860, "queue in"=w8862) -> ("error out"=w8858:errorcluster)  [unwired: 7 in, 1 out]
        }
        n4074 = Merge Errors(w8823, w8822) -> (w8821:errorcluster)
      }
      frame "Test DRV 50A" {
        w8870 = T11 {"command"="", "command data"=variant} ("element")
        w8864 = 50 ("DUT index(0-59)")
        w8896 = T11 {"command"="", "command data"=variant} ("element")
        n4075 = disable-structure shown="LOGGING==TRUE" {
          disable-tunnel: w8874 -> [w8911 _]
          frame condition #0 (active) {
            n4076 = Empty String/Path?(string/path=w8911) -> (empty?=w8914:bool)
            n4077 = Select(t="Quece timeout", s=w8914, f=w8911) -> (s? t:f=w8910:string)
            n4078 = call "string log (SubVI).vi"("Enum"=enum16{"Init", "Log", "Read"}."Log", "state Name"=w8910) -> ()  [unwired: 8 in, 2 out]
          }
          frame condition #1 {
          }
        }
        n4079 = Flush Queue(queue=w8875) -> (queue out=w8876:refnum<queue>)  [unwired: 1 in, 2 out]
        n4080 = Decrement(x=w8864) -> (x-1=w8867:i32)
        n4081 = Index Array(array=w8865, index=w8867) -> (element=w8863:refnum<vi>)
        n4082 = property class="ColBox"(reference=w8863, "Value"=u32 10000536 ("DRV 1")) -> ()  [unwired: 1 in, 2 out]
        n4083 = To Variant(anything=bool[] [FALSE, TRUE, FALSE, FALSE, FALSE, FALSE]) -> (Variant=w8893:variant)
        n4084 = To Variant(anything=T6."demux1_10_channel9" ("demux1_10(x6)_encode")) -> (Variant=w8897:variant)
        n4085 = To Variant(anything=T4."mux6_1_channel2_3" ("mux6_1(3wires)_encode")) -> (Variant=w8900:variant)
        n4086 = To Variant(anything=T5."mux10_1_channel9" ("mux10_1(x6)_encode")) -> (Variant=w8902:variant)
        n4087 = Bundle By Name(cluster=w8896, "command"="MEAS.mux10-1", "command data"=w8902) -> (w8891:T11)
        n4088 = Bundle By Name(cluster=w8896, "command"="MEAS.mux6_1", "command data"=w8900) -> (w8890:T11)
        n4089 = Bundle By Name(cluster=w8896, "command"="MEAS.demux1-10", "command data"=w8897) -> (w8889:T11)
        n4090 = Bundle By Name(cluster=w8896, "command"="MEAS.eMIC", "command data"=w8893) -> (w8888:T11)
        n4091 = Bundle By Name(cluster=w8896, "command"="MEAS.AllRelaysOFF") -> (w8892:T11)
        n4092 = Build Array(w8892, w8891, w8890, w8889, w8888) -> (w8883:T11[])
        n4093 = Bundle By Name(cluster=w8870, "command"="MEAS.requestAC", "command data"=w8864) -> (w8884:T11)
        n4094 = Bundle By Name(cluster=w8870, "command"="Apps.WaitForEvent", "command data"=w8864) -> (w8869:T11)
        n4095 = Bundle By Name(cluster=w8870, "command"="MEAS.DMM dual read") -> (w8885:T11)
        n4096 = Bundle By Name(cluster=w8870, "command"="Apps.UI Update 1") -> (w8871:T11)
        n4097 = Build Array(w8885, w8884, w8869, w8871) -> (w8882:T11[])
        n4098 = Build Array (concatenate)(w8883, w8882) -> (w8881:T11[])
        n4099 = for {
          tunnel: w8881 -> [w8918] mode=indexing
          tunnel: w8876 -> [w8919]
          tunnel: [w8915] -> w8879 mode=indexing
          n4100 = Unbundle By Name(w8918) -> ("command"=w8917:string, "command data"=w8916:variant)
          n4101 = call "App enquece.vi"("command data"=w8916, "command"=w8917, "queue in"=w8919) -> ("error out"=w8915:errorcluster)  [unwired: 7 in, 1 out]
        }
        n4102 = Merge Errors(w8880, w8879) -> (w8878:errorcluster)
      }
      frame "Test DRV 51A" {
        w8927 = T11 {"command"="", "command data"=variant} ("element")
        w8920 = 51 ("DUT index(0-59)")
        w8953 = T11 {"command"="", "command data"=variant} ("element")
        n4103 = disable-structure shown="LOGGING==TRUE" {
          disable-tunnel: w8931 -> [w8968 _]
          frame condition #0 (active) {
            n4104 = Empty String/Path?(string/path=w8968) -> (empty?=w8971:bool)
            n4105 = Select(t="Quece timeout", s=w8971, f=w8968) -> (s? t:f=w8967:string)
            n4106 = call "string log (SubVI).vi"("Enum"=enum16{"Init", "Log", "Read"}."Log", "state Name"=w8967) -> ()  [unwired: 8 in, 2 out]
          }
          frame condition #1 {
          }
        }
        n4107 = Flush Queue(queue=w8932) -> (queue out=w8933:refnum<queue>)  [unwired: 1 in, 2 out]
        n4108 = Decrement(x=w8920) -> (x-1=w8924:i32)
        n4109 = Index Array(array=w8921, index=w8924) -> (element=w8922:refnum<vi>)
        n4110 = property class="ColBox"(reference=w8922, "Value"=u32 10000536 ("DRV 1")) -> ()  [unwired: 1 in, 2 out]
        n4111 = To Variant(anything=bool[] [FALSE, FALSE, TRUE, FALSE, FALSE, FALSE]) -> (Variant=w8950:variant)
        n4112 = To Variant(anything=T6."demux1_10_channel9" ("demux1_10(x6)_encode")) -> (Variant=w8954:variant)
        n4113 = To Variant(anything=T4."mux6_1_channel3_3" ("mux6_1(3wires)_encode")) -> (Variant=w8957:variant)
        n4114 = To Variant(anything=T5."mux10_1_channel9" ("mux10_1(x6)_encode")) -> (Variant=w8959:variant)
        n4115 = Bundle By Name(cluster=w8953, "command"="MEAS.mux10-1", "command data"=w8959) -> (w8948:T11)
        n4116 = Bundle By Name(cluster=w8953, "command"="MEAS.mux6_1", "command data"=w8957) -> (w8947:T11)
        n4117 = Bundle By Name(cluster=w8953, "command"="MEAS.demux1-10", "command data"=w8954) -> (w8946:T11)
        n4118 = Bundle By Name(cluster=w8953, "command"="MEAS.eMIC", "command data"=w8950) -> (w8945:T11)
        n4119 = Bundle By Name(cluster=w8953, "command"="MEAS.AllRelaysOFF") -> (w8949:T11)
        n4120 = Build Array(w8949, w8948, w8947, w8946, w8945) -> (w8940:T11[])
        n4121 = Bundle By Name(cluster=w8927, "command"="MEAS.requestAC", "command data"=w8920) -> (w8941:T11)
        n4122 = Bundle By Name(cluster=w8927, "command"="Apps.WaitForEvent", "command data"=w8920) -> (w8926:T11)
        n4123 = Bundle By Name(cluster=w8927, "command"="MEAS.DMM dual read") -> (w8942:T11)
        n4124 = Bundle By Name(cluster=w8927, "command"="Apps.UI Update 1") -> (w8928:T11)
        n4125 = Build Array(w8942, w8941, w8926, w8928) -> (w8939:T11[])
        n4126 = Build Array (concatenate)(w8940, w8939) -> (w8938:T11[])
        n4127 = for {
          tunnel: w8938 -> [w8975] mode=indexing
          tunnel: w8933 -> [w8976]
          tunnel: [w8972] -> w8936 mode=indexing
          n4128 = Unbundle By Name(w8975) -> ("command"=w8974:string, "command data"=w8973:variant)
          n4129 = call "App enquece.vi"("command data"=w8973, "command"=w8974, "queue in"=w8976) -> ("error out"=w8972:errorcluster)  [unwired: 7 in, 1 out]
        }
        n4130 = Merge Errors(w8937, w8936) -> (w8935:errorcluster)
      }
      frame "Test DRV 52A" {
        w8984 = T11 {"command"="", "command data"=variant} ("element")
        w8977 = 52 ("DUT index(0-59)")
        w9010 = T11 {"command"="", "command data"=variant} ("element")
        n4131 = disable-structure shown="LOGGING==TRUE" {
          disable-tunnel: w8988 -> [w9025 _]
          frame condition #0 (active) {
            n4132 = Empty String/Path?(string/path=w9025) -> (empty?=w9028:bool)
            n4133 = Select(t="Quece timeout", s=w9028, f=w9025) -> (s? t:f=w9024:string)
            n4134 = call "string log (SubVI).vi"("Enum"=enum16{"Init", "Log", "Read"}."Log", "state Name"=w9024) -> ()  [unwired: 8 in, 2 out]
          }
          frame condition #1 {
          }
        }
        n4135 = Flush Queue(queue=w8989) -> (queue out=w8990:refnum<queue>)  [unwired: 1 in, 2 out]
        n4136 = Decrement(x=w8977) -> (x-1=w8981:i32)
        n4137 = Index Array(array=w8978, index=w8981) -> (element=w8979:refnum<vi>)
        n4138 = property class="ColBox"(reference=w8979, "Value"=u32 10000536 ("DRV 1")) -> ()  [unwired: 1 in, 2 out]
        n4139 = To Variant(anything=bool[] [FALSE, FALSE, FALSE, TRUE, FALSE, FALSE]) -> (Variant=w9007:variant)
        n4140 = To Variant(anything=T6."demux1_10_channel9" ("demux1_10(x6)_encode")) -> (Variant=w9011:variant)
        n4141 = To Variant(anything=T4."mux6_1_channel4_3" ("mux6_1(3wires)_encode")) -> (Variant=w9014:variant)
        n4142 = To Variant(anything=T5."mux10_1_channel9" ("mux10_1(x6)_encode")) -> (Variant=w9016:variant)
        n4143 = Bundle By Name(cluster=w9010, "command"="MEAS.mux10-1", "command data"=w9016) -> (w9005:T11)
        n4144 = Bundle By Name(cluster=w9010, "command"="MEAS.mux6_1", "command data"=w9014) -> (w9004:T11)
        n4145 = Bundle By Name(cluster=w9010, "command"="MEAS.demux1-10", "command data"=w9011) -> (w9003:T11)
        n4146 = Bundle By Name(cluster=w9010, "command"="MEAS.eMIC", "command data"=w9007) -> (w9002:T11)
        n4147 = Bundle By Name(cluster=w9010, "command"="MEAS.AllRelaysOFF") -> (w9006:T11)
        n4148 = Build Array(w9006, w9005, w9004, w9003, w9002) -> (w8997:T11[])
        n4149 = Bundle By Name(cluster=w8984, "command"="MEAS.requestAC", "command data"=w8977) -> (w8998:T11)
        n4150 = Bundle By Name(cluster=w8984, "command"="Apps.WaitForEvent", "command data"=w8977) -> (w8983:T11)
        n4151 = Bundle By Name(cluster=w8984, "command"="MEAS.DMM dual read") -> (w8999:T11)
        n4152 = Bundle By Name(cluster=w8984, "command"="Apps.UI Update 1") -> (w8985:T11)
        n4153 = Build Array(w8999, w8998, w8983, w8985) -> (w8996:T11[])
        n4154 = Build Array (concatenate)(w8997, w8996) -> (w8995:T11[])
        n4155 = for {
          tunnel: w8995 -> [w9032] mode=indexing
          tunnel: w8990 -> [w9033]
          tunnel: [w9029] -> w8993 mode=indexing
          n4156 = Unbundle By Name(w9032) -> ("command"=w9031:string, "command data"=w9030:variant)
          n4157 = call "App enquece.vi"("command data"=w9030, "command"=w9031, "queue in"=w9033) -> ("error out"=w9029:errorcluster)  [unwired: 7 in, 1 out]
        }
        n4158 = Merge Errors(w8994, w8993) -> (w8992:errorcluster)
      }
      frame "Test DRV 53A" {
        w9042 = T11 {"command"="", "command data"=variant} ("element")
        w9034 = 53 ("DUT index(0-59)")
        w9067 = T11 {"command"="", "command data"=variant} ("element")
        n4159 = disable-structure shown="LOGGING==TRUE" {
          disable-tunnel: w9046 -> [w9082 _]
          frame condition #0 (active) {
            n4160 = Empty String/Path?(string/path=w9082) -> (empty?=w9085:bool)
            n4161 = Select(t="Quece timeout", s=w9085, f=w9082) -> (s? t:f=w9081:string)
            n4162 = call "string log (SubVI).vi"("Enum"=enum16{"Init", "Log", "Read"}."Log", "state Name"=w9081) -> ()  [unwired: 8 in, 2 out]
          }
          frame condition #1 {
          }
        }
        n4163 = Flush Queue(queue=w9047) -> (queue out=w9048:refnum<queue>)  [unwired: 1 in, 2 out]
        n4164 = Decrement(x=w9034) -> (x-1=w9038:i32)
        n4165 = Index Array(array=w9035, index=w9038) -> (element=w9036:refnum<vi>)
        n4166 = property class="ColBox"(reference=w9036, "Value"=u32 10000536 ("DRV 1")) -> ()  [unwired: 1 in, 2 out]
        n4167 = To Variant(anything=bool[] [FALSE, FALSE, FALSE, FALSE, TRUE, FALSE]) -> (Variant=w9064:variant)
        n4168 = To Variant(anything=T6."demux1_10_channel9" ("demux1_10(x6)_encode")) -> (Variant=w9068:variant)
        n4169 = To Variant(anything=T4."mux6_1_channel5_3" ("mux6_1(3wires)_encode")) -> (Variant=w9071:variant)
        n4170 = To Variant(anything=T5."mux10_1_channel9" ("mux10_1(x6)_encode")) -> (Variant=w9073:variant)
        n4171 = Bundle By Name(cluster=w9067, "command"="MEAS.mux10-1", "command data"=w9073) -> (w9062:T11)
        n4172 = Bundle By Name(cluster=w9067, "command"="MEAS.mux6_1", "command data"=w9071) -> (w9061:T11)
        n4173 = Bundle By Name(cluster=w9067, "command"="MEAS.demux1-10", "command data"=w9068) -> (w9060:T11)
        n4174 = Bundle By Name(cluster=w9067, "command"="MEAS.eMIC", "command data"=w9064) -> (w9059:T11)
        n4175 = Bundle By Name(cluster=w9067, "command"="MEAS.AllRelaysOFF") -> (w9063:T11)
        n4176 = Build Array(w9063, w9062, w9061, w9060, w9059) -> (w9055:T11[])
        n4177 = Bundle By Name(cluster=w9042, "command"="MEAS.requestAC", "command data"=w9034) -> (w9056:T11)
        n4178 = Bundle By Name(cluster=w9042, "command"="Apps.WaitForEvent", "command data"=w9034) -> (w9041:T11)
        n4179 = Bundle By Name(cluster=w9042, "command"="MEAS.DMM dual read") -> (w9057:T11)
        n4180 = Bundle By Name(cluster=w9042, "command"="Apps.UI Update 1") -> (w9043:T11)
        n4181 = Build Array(w9057, w9056, w9041, w9043) -> (w9054:T11[])
        n4182 = Build Array (concatenate)(w9055, w9054) -> (w9053:T11[])
        n4183 = for {
          tunnel: w9053 -> [w9089] mode=indexing
          tunnel: w9048 -> [w9090]
          tunnel: [w9086] -> w9051 mode=indexing
          n4184 = Unbundle By Name(w9089) -> ("command"=w9088:string, "command data"=w9087:variant)
          n4185 = call "App enquece.vi"("command data"=w9087, "command"=w9088, "queue in"=w9090) -> ("error out"=w9086:errorcluster)  [unwired: 7 in, 1 out]
        }
        n4186 = Merge Errors(w9052, w9051) -> (w9050:errorcluster)
      }
      frame "Test DRV 54A" {
        w9098 = T11 {"command"="", "command data"=variant} ("element")
        w9091 = 54 ("DUT index(0-59)")
        w9124 = T11 {"command"="", "command data"=variant} ("element")
        n4187 = disable-structure shown="LOGGING==TRUE" {
          disable-tunnel: w9102 -> [w9139 _]
          frame condition #0 (active) {
            n4188 = Empty String/Path?(string/path=w9139) -> (empty?=w9142:bool)
            n4189 = Select(t="Quece timeout", s=w9142, f=w9139) -> (s? t:f=w9138:string)
            n4190 = call "string log (SubVI).vi"("Enum"=enum16{"Init", "Log", "Read"}."Log", "state Name"=w9138) -> ()  [unwired: 8 in, 2 out]
          }
          frame condition #1 {
          }
        }
        n4191 = Flush Queue(queue=w9103) -> (queue out=w9104:refnum<queue>)  [unwired: 1 in, 2 out]
        n4192 = Decrement(x=w9091) -> (x-1=w9095:i32)
        n4193 = Index Array(array=w9092, index=w9095) -> (element=w9093:refnum<vi>)
        n4194 = property class="ColBox"(reference=w9093, "Value"=u32 10000536 ("DRV 1")) -> ()  [unwired: 1 in, 2 out]
        n4195 = To Variant(anything=bool[] [FALSE, FALSE, FALSE, FALSE, FALSE, TRUE]) -> (Variant=w9121:variant)
        n4196 = To Variant(anything=T6."demux1_10_channel9" ("demux1_10(x6)_encode")) -> (Variant=w9125:variant)
        n4197 = To Variant(anything=T4."mux6_1_channel6_3" ("mux6_1(3wires)_encode")) -> (Variant=w9128:variant)
        n4198 = To Variant(anything=T5."mux10_1_channel9" ("mux10_1(x6)_encode")) -> (Variant=w9130:variant)
